vi "AviFrameReader.vi"() -> ()   [LabVIEW 2013]
uses:
  <vilib>/vision/Avi.llb/IMAQ AVI2 Codec Path.ctl
panel:
  in  "stop":bool
  in  "Frame Number":u32
  out "Image":T1(plugin-control)
  in  "AVI File Path":path
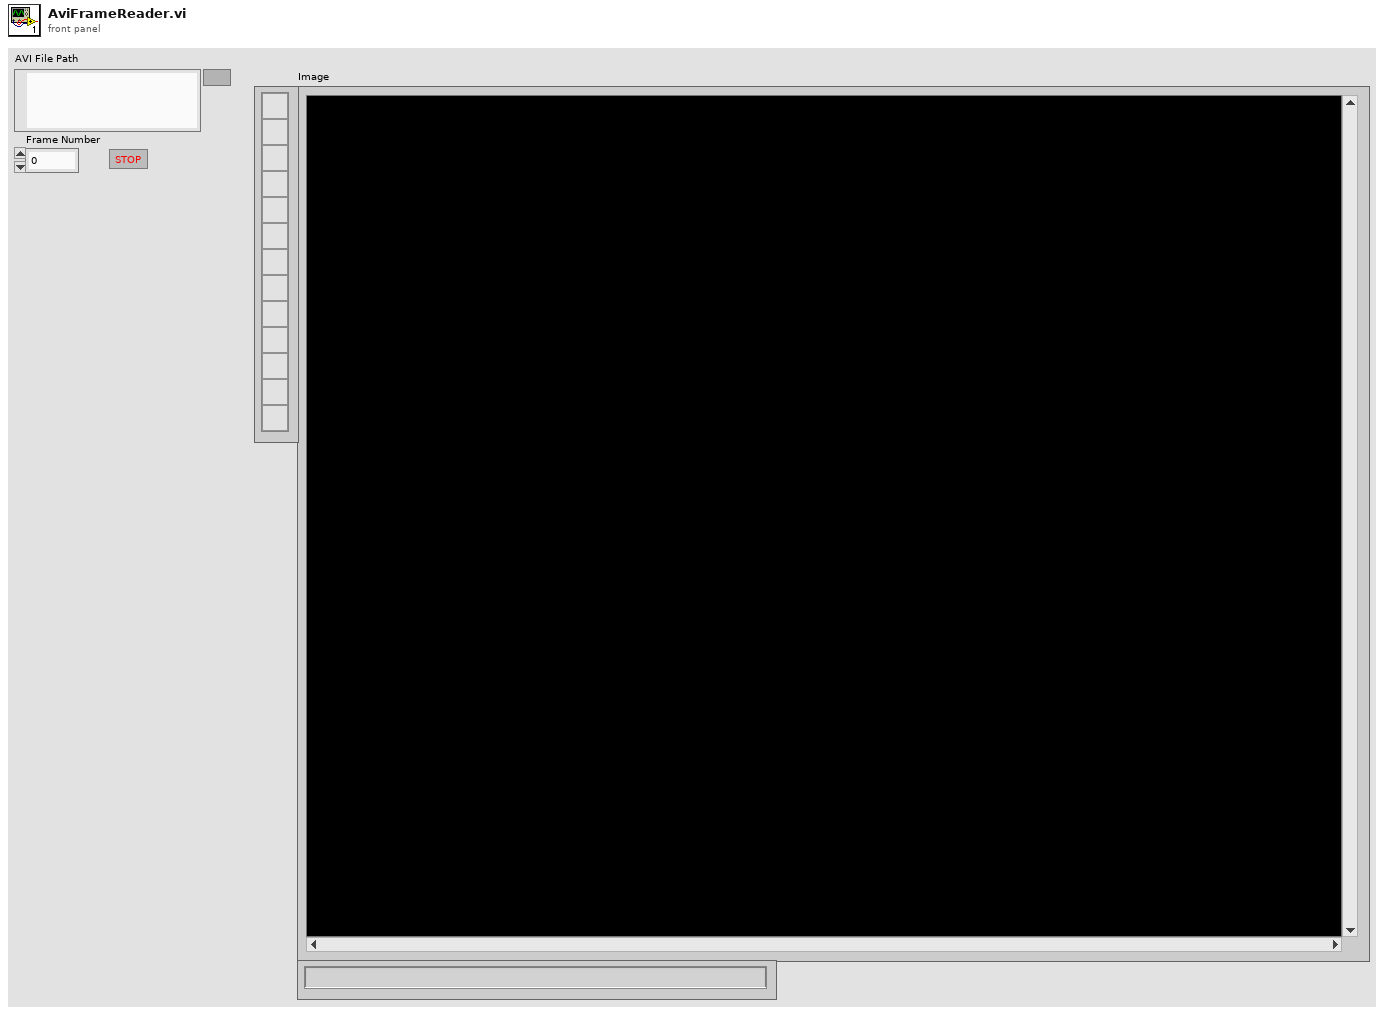
[diagram p1: front panel]
types:
  T1 = typedef "IMAQ Image.ctl" = refnum<image>
  T2 = typedef "IMAQ AVI2 Codec Path.ctl" = u32
  T3 = typedef "IMAQ AVI2 Refnum.ctl" = refnum<k20>
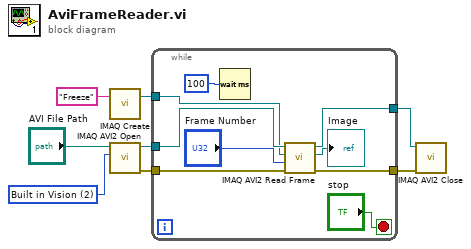
[diagram p0: block diagram]
diagram:
  w5 = T2 2 items=["Default", "System", "Built in Vision"] ("Codec Source")
  n1 = call "IMAQ Create"("Image Name"="Freeze") -> ("New Image"=w3:T1)  [unwired: 4 in, 1 out]
  n2 = call "IMAQ AVI2 Open"("Codec Source"=w5, "AVI File Path"="AVI File Path") -> ("error out"=w6:errorcluster, "AVI Refnum"=w7:T3)  [unwired: 8 in]
  n3 = while {
    tunnel: w7 -> [w17]
    tunnel: w6 -> [w16]
    tunnel: w3 -> [w14]
    tunnel: [w11] -> w2
    tunnel: [w10] -> w1
    stop <- "stop" stop-if-true
    n4 = Wait (ms)(milliseconds to wait=u32 100) -> ()  [unwired: 1 out]
    n5 = call "IMAQ AVI2 Read Frame"("error in (no error)"=w16, "Frame Number"="Frame Number", "Image"=w14, "AVI Refnum"=w17) -> ("error out"=w10:errorcluster, "Image Out"=→"Image":T1, "AVI Refnum (duplicate)"=w11:T3)  [unwired: 5 in]
  }
  n6 = call "IMAQ AVI2 Close"("error in (no error)"=w1, "AVI Refnum"=w2) -> ()  [unwired: 9 in, 1 out]
